vi "CVT to JSON.vi"(8 "error in":errorcluster, 11 "cvt":refnum<data-value>) -> (0 "error out":errorcluster, 2 "json cvt":string, 3 "cvt 2":refnum<data-value>)   [LabVIEW 2014]
uses:
  <userlib>/_OpenG.lib/lvdata/lvdata.llb/Type Descriptor Enumeration__ogtk.ctl
panel:
  out "Array":T1[](array[typedef]) format="%.0x"
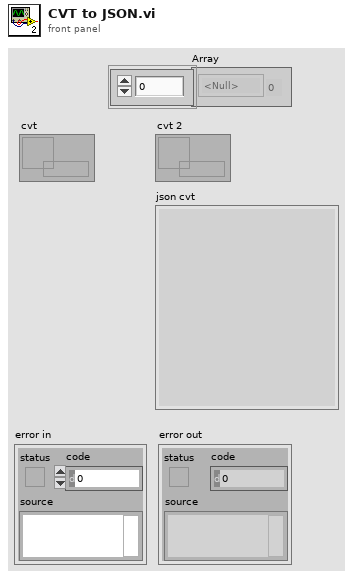
[diagram p1: front panel]
types:
  T1 = typedef "Type Descriptor Enumeration__ogtk.ctl" = enum8{"<Null>", "I8", "I16", "I32", "I64", "U8", "U16", "U32", "U64", "SGL", "DBL", "EXT", "CSG", "CDB", "CXT", "0x0F", "0x10", "0x11", "0x12", "0x13", "0x14", "Enum U8", "Enum U16", "Enum U32", "Enum U64", "SGL PQ", "DBL PQ", "EXT PQ", "CSG PQ", "CDB PQ", "CXT PQ", "0x1F", "0x20", "Boolean", "0x22", "0x23", "0x24", "0x25", "0x26", "0x27", "0x28", "0x29", "0x2A", "0x2B", "0x2C", "0x2D", "0x2E", "0x2F", "String", "0x31", "Path", "Pict", "0x34", "0x35", "0x36", "DAQ", "0x38", "0x39", "0x3A", "0x3B", "0x3C", "0x3D", "0x3E", "0x3F", "Array", "0x41", "0x42", "0x43", "0x44", "0x45", "0x46", "0x47", "0x48", "0x49", "0x4A", "0x4B", "0x4C", "0x4D", "0x4E", "0x4F", "Cluster", "0x51", "0x52", "Variant", "Waveform", "0x55", "0x56", "0x57", "0x58", "0x59", "0x5A", "0x5B", "0x5C", "0x5D", "0x5E", "0x5F", "0x60", "0x61", "0x62", "0x63", "0x64", "0x65", "0x66", "0x67", "0x68", "0x69", "0x6A", "0x6B", "0x6C", "0x6D", "0x6E", "0x6F", "Refnum"}
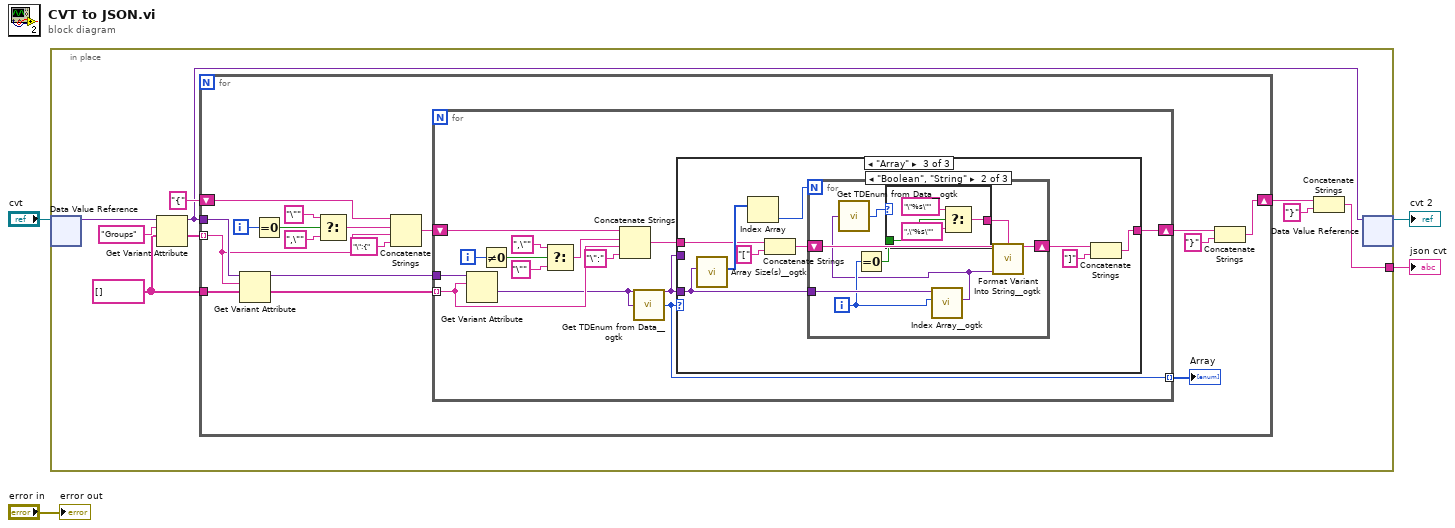
[diagram p0: block diagram]
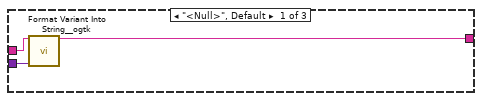
[diagram p2: hidden frame]
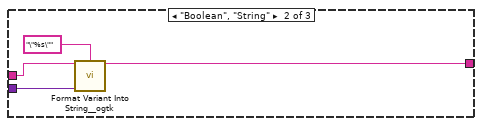
[diagram p3: hidden frame]
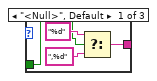
[diagram p4: hidden frame]
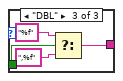
[diagram p5: hidden frame]
diagram:
  n1 = in-place {
    in-place-border: [w5] -> w3
    w10 = string[] []
    n2 = in-place-dvr #1("cvt") -> (w13:variant)  [unwired: 1 out]
    n3 = Get Variant Attribute(Variant=w13, name="Groups", default value (empty Variant)=w10) -> (duplicate Variant=w6:variant, value=w11:string[])  [unwired: 1 in, 2 out]
    n4 = for {
      tunnel: w6 -> [w30]
      tunnel: w11 -> [w25] mode=indexing
      tunnel: w10 -> [w29]
      shift-right: [w15] -> w8
      shift-left: "{" -> [w26]
      i -> [w22]
      n5 = Get Variant Attribute(Variant=w30, name=w25, default value (empty Variant)=w29) -> (duplicate Variant=w27:variant, value=w28:string[])  [unwired: 1 in, 2 out]
      n6 = Equal To 0?(x=w22) -> (x = 0?=w21:bool)
      n7 = Select(t="\"" ("string"), s=w21, f=",\"" ("string")) -> (s? t:f=w18:string)
      n8 = Concatenate Strings(w26, w18, w25, "\":{" ("string")) -> (w23:string)
      n9 = for {
        tunnel: w28 -> [w42] mode=indexing
        tunnel: w27 -> [w43]
        shift-right: [w32] -> w17
        shift-left: w23 -> [w40]
        tunnel: [w34] -> w14 mode=indexing
        i -> [w39]
        n10 = Get Variant Attribute(Variant=w43, name=w42) -> (value=w33:variant)  [unwired: 2 in, 3 out]
        n11 = Not Equal To 0?(x=w39) -> (x != 0?=w38:bool)
        n12 = Select(t=",\"" ("string"), s=w38, f="\"" ("string")) -> (s? t:f=w35:string)
        n13 = Concatenate Strings(w40, w35, w42, "\":" ("string")) -> (w31:string)
        n14 = call <userlib>:"Get TDEnum from Data__ogtk.vi"("Data"=w33) -> ("Type Descriptor Enumeration"=w34:T1)  [unwired: 4 in]
        n15 = case shown="\"Array\"" w34 {
          tunnel: w33 -> [_ _ w57]
          tunnel: w33 -> [w46 w50 _]
          tunnel: [w45 w47 w52] -> w32
          tunnel: w31 -> [w44 w48 w56]
          frame "<Null>", Default {
            n16 = call <userlib>:"Format Variant Into String__ogtk.vi"("Input String"=w44, "Variant"=w46) -> ("Output String"=w45:string)  [unwired: 12 in, 1 out]
          }
          frame "Boolean", "String" {
            n17 = call <userlib>:"Format Variant Into String__ogtk.vi"("Input String"=w48, "Format String"="\"%s\"", "Variant"=w50) -> ("Output String"=w47:string)  [unwired: 11 in, 1 out]
          }
          frame "Array" {
            n18 = call <userlib>:"Array Size(s)__ogtk.vi"("Array"=w57) -> ("Size(s)"=w59:u32[])  [unwired: 8 in, 2 out]
            n19 = Index Array(array=w59) -> (element=w58:u32)  [unwired: 1 in]
            n20 = Concatenate Strings(w56, "[" ("string")) -> (w54:string)
            n21 = for {
              N: w58 -> [_]
              tunnel: w57 -> [w67]
              shift-right: [w62] -> w53
              shift-left: w54 -> [w66]
              i -> [w65]
              n22 = Equal To 0?(x=w65) -> (x = 0?=w64:bool)
              n23 = call <userlib>:"Index Array__ogtk.vi"("Index (1D)"=w65, "MultiD Array"=w67) -> ("Array Element"=w61:variant)  [unwired: 8 in, 1 out]
              n24 = call <userlib>:"Get TDEnum from Data__ogtk.vi"("Data"=w61) -> ("Type Descriptor Enumeration"=w60:T1)  [unwired: 4 in]
              n25 = case shown="\"Boolean\", \"String\"" w60 {
                tunnel: w64 -> [w68 w73 w79]
                tunnel: [w69 w72 w76] -> w63
                frame "<Null>", Default {
                  n26 = Select(t="%d", s=w68, f=",%d") -> (s? t:f=w69:string)
                }
                frame "Boolean", "String" {
                  n27 = Select(t="\"%s\"", s=w73, f=",\"%s\"") -> (s? t:f=w72:string)
                }
                frame "DBL" {
                  n28 = Select(t="%f", s=w79, f=",%f") -> (s? t:f=w76:string)
                }
              }
              n29 = call <userlib>:"Format Variant Into String__ogtk.vi"("Input String"=w66, "Format String"=w63, "Variant"=w61) -> ("Output String"=w62:string)  [unwired: 11 in, 1 out]
            }
            n30 = Concatenate Strings(w53, "]" ("string")) -> (w52:string)
          }
        }
      }
      "Array" <- w14
      n31 = Concatenate Strings(w17, "}" ("string")) -> (w15:string)
    }
    n32 = Concatenate Strings(w8, "}" ("string")) -> (w5:string)
    n33 = in-place-dvr #1(w6) -> (→"cvt 2":refnum<data-value>)  [unwired: 1 out]
  }
  "json cvt" <- w3
  "error out" <- "error in"
